vi "Add time to filename base.vi"(4 "Filename base":string="abc", 5 "Include msec?":bool) -> (1 "String+time":string="abc_2007-07-20_094157")   [LabVIEW 2010]
doc: "Appends date and time strings to filename. If include msec? = T adds underscore and msec."
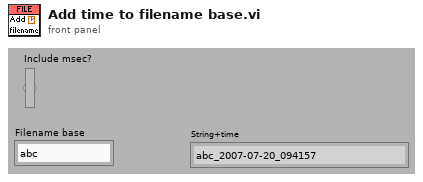
[diagram p1: front panel]
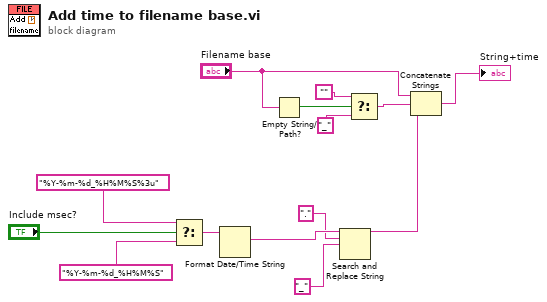
[diagram p0: block diagram]
diagram:
  n1 = Select(t="%Y-%m-%d_%H%M%S%3u" ("time format string (%c)"), s="Include msec?", f="%Y-%m-%d_%H%M%S" ("time format string (%c)")) -> (s? t:f=w6:string)
  n2 = Format Date/Time String(time format string (%c)=w6) -> (date/time string=w4:string)  [unwired: 2 out]
  n3 = Empty String/Path?(string/path="Filename base") -> (empty?=w11:bool)
  n4 = Search and Replace String(input string=w4, search string=".", replace string="_" ("replace string (\"\")")) -> (result string=w1:string)  [unwired: 1 in, 7 out]
  n5 = Select(t="", s=w11, f="_" ("string")) -> (s? t:f=w14:string)
  n6 = Concatenate Strings("Filename base", w14, w1) -> (→"String+time":string)
